vi "Find all vis in memory with duplicate documentation.vi"() -> ()   [LabVIEW 2010]
doc: "This .vi searches all .vi's in memory and returns the ones that have duplicate documentation. The .vis that are controls, in the .vi lib are ignored. The control on the front panel allows these .vis to be openned."
panel:
  out "Total # with duplicate doc":i32
  out "Files with duplicate \nDocumentation":path[](array[path])
  out "Vis checked":i32(slide) scale=0.0..1965.0
  in  "Open FPs?":bool caption="Open FPs of VI's without Documentation?"
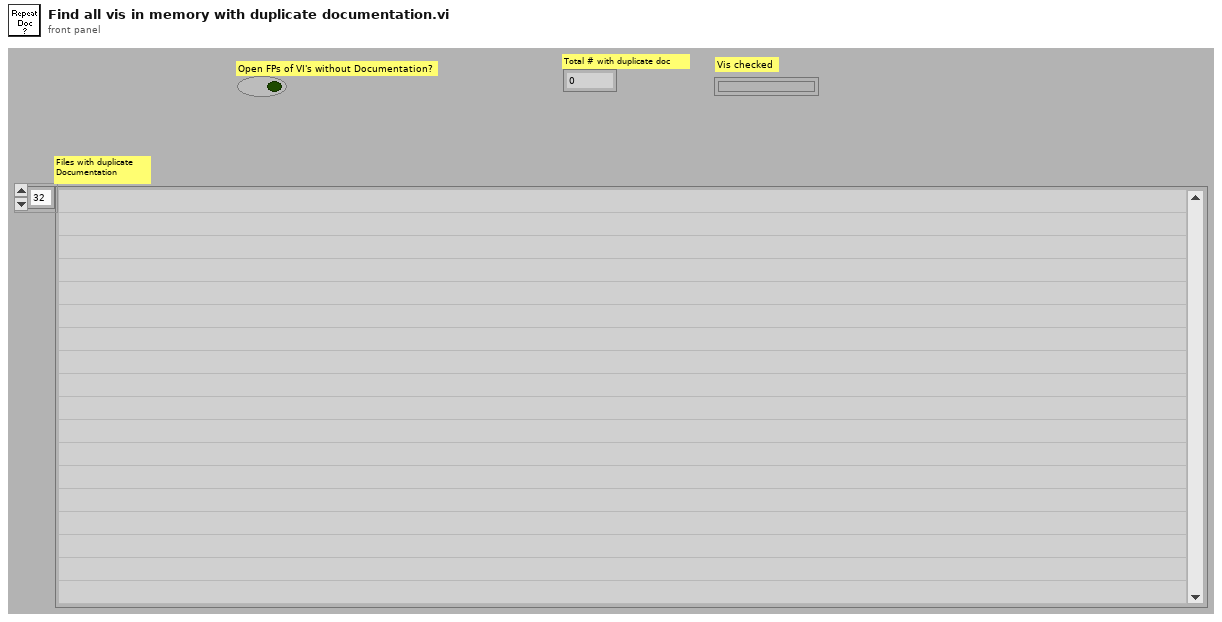
[diagram p1: front panel]
types:
  T1 = enum32{"invalid VI type", "Standard VI", "Control VI", "Global VI", "Polymorphic VI", "Configuration VI", "SubSystem", "Facade VI", "Method VI", "Statechart Diagram VI"}
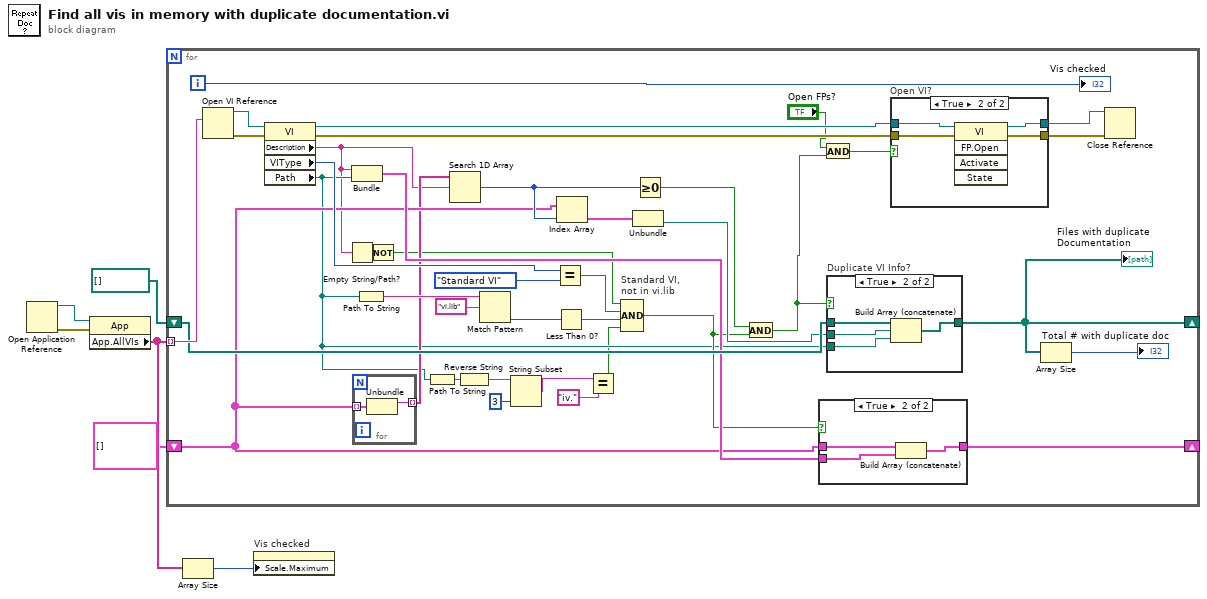
[diagram p0: block diagram]
diagram:
  n1 = Open Application Reference() -> (0:w5:errorcluster, 3:w6:refnum<vi>)  [unwired: 1 in, 3 out]
  n2 = property class="App"(reference=w6, error in=w5) -> ("App.AllVIs"=w4:string[])  [unwired: 2 out]
  n3 = for {
    tunnel: w4 -> [w42] mode=indexing
    shift-right: [w30] -> _
    shift-left: cluster{"Description":string, "Path":path}[] [] -> [w23]
    shift-right: [w7] -> _
    shift-left: path[] [] -> [w29]
    i -> [w31]
    n4 = Open VI Reference(vi path=w42) -> (vi reference=w46:refnum<vi>, error out=w45:errorcluster)  [unwired: 1 in, 4 out]
    n5 = property class="VI"(reference=w46, error in=w45) -> (reference out=w37:refnum<vi>, error out=w36:errorcluster, "Description"=w10:string, "VIType"=w44:T1, "Path"=w16:path)
    n6 = Empty String/Path?(string/path=w10) -> (empty?=w9:bool)
    n7 = Bundle("Description"=w10, "Path"=w16) -> (w24:cluster{"Description":string, "Path":path})  [unwired: 1 out]
    n8 = for {
      tunnel: w23 -> [w48] mode=indexing
      tunnel: [w47] -> w22 mode=indexing
      n9 = Unbundle(w48) -> ("Description"=w47:string)  [unwired: 1 out]
    }
    n10 = Path To String(path=w16) -> (string=w38:string)
    n11 = Not(x=w9) -> (.not. x?=w8:bool)
    n12 = Path To String(path=w16) -> (string=w15:string)
    n13 = Search 1D Array(1D array=w22, element=w10) -> (index of element=w28:i32)  [unwired: 1 out]
    n14 = Reverse String(1:w15) -> (0:w13:string)
    n15 = Match Pattern(string=w38, regular expression="vi.lib") -> (offset past match=w40:i32)  [unwired: 4 out]
    n16 = String Subset(string=w13, length (rest)=3 ("length (rest)")) -> (substring=w12:string)  [unwired: 1 out]
    n17 = Equal?(x=w44, y=T1."Standard VI" ("VI Type")) -> (x = y?=w32:bool)
    n18 = Less Than 0?(x=w40) -> (x < 0?=w39:bool)
    n19 = Index Array(array=w23, index=w28) -> (element=w21:cluster{"Description":string, "Path":path})
    n20 = Equal?(x=w12, y="iv.") -> (x = y?=w14:bool)
    n21 = Compound Arithmetic op=AND "Standard VI,\nnot in vi.lib"(w8, w32, w39, w14) -> (w19:bool)
    n22 = Unbundle(w21) -> ("Path"=w20:path)  [unwired: 1 out]
    n23 = Greater Or Equal To 0?(x=w28) -> (x >= 0?=w27:bool)
    n24 = And(x=w27, y=w19) -> (x .and. y?=w18:bool)
    n25 = case shown="True" w19 {
      tunnel: [w49 w50] -> w30
      tunnel: w23 -> [w49 w52]
      tunnel: w24 -> [_ w51]
      frame False {
      }
      frame True {
        n26 = Build Array (concatenate)(w52, w51) -> (w50:cluster{"Description":string, "Path":path}[])
      }
    }
    n27 = And(x="Open FPs?", y=w18) -> (x .and. y?=w33:bool)
    n28 = case "Duplicate VI Info?" shown="True" w18 {
      tunnel: w20 -> [_ w55]
      tunnel: [w53 w57] -> w7
      tunnel: w29 -> [w53 w56]
      tunnel: w16 -> [_ w54]
      frame False {
      }
      frame True {
        n29 = Build Array (concatenate)(w56, w55, w54) -> (w57:path[])
      }
    }
    "Files with duplicate \nDocumentation" <- w7
    n30 = case "Open VI?" shown="True" w33 {
      tunnel: w37 -> [w58 w63]
      tunnel: w36 -> [w59 w62]
      tunnel: [w58 w61] -> w35
      tunnel: [w59 w60] -> w34
      frame False {
      }
      frame True {
        n31 = invoke class="VI" method="FP.Open"(reference=w63, error in=w62) -> (reference out=w61:refnum<vi>, error out=w60:errorcluster)  [unwired: 3 in, 3 out]
      }
    }
    n32 = Array Size(array=w7) -> (size(s)=→"Total # with duplicate doc":i32)
    n33 = Close Reference(reference=w35, error in (no error)=w34) -> ()  [unwired: 1 out]
    "Vis checked" <- w31
  }
  n34 = Array Size(array=w4) -> (size(s)=w3:i32)
  n35 = property on="Vis checked" class="Slide (strict)"("Scale.Maximum"=w3) -> ()  [unwired: 2 in, 2 out]
